vi "Plus minus conditional.vi"(8 "Percent Floor":dbl=2.0, 9 "Actual Number":dbl, 10 "Target":dbl, 11 "Percent ceiling":dbl=2.0) -> (0 "Below":bool, 2 "Either":bool, 3 "Above":bool)   [LabVIEW 2012]
doc: "This VI check to see if a number is above or below a certain percent."
panel:
  out "min":dbl
  out "max":dbl
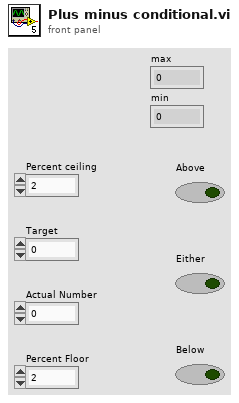
[diagram p1: front panel]
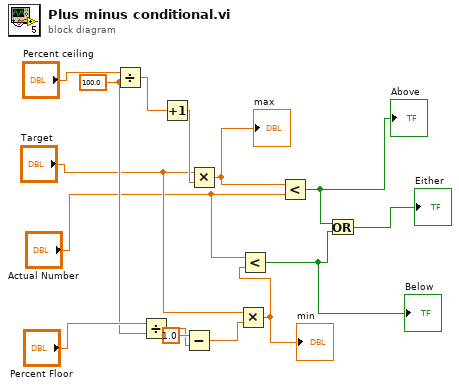
[diagram p0: block diagram]
diagram:
  w13 = 100.0 ("y")
  n1 = Divide(x="Percent ceiling", y=w13) -> (x/y=w12:dbl)
  n2 = Divide(x="Percent Floor", y=w13) -> (x/y=w2:dbl)
  n3 = Increment(x=w12) -> (x+1=w11:dbl)
  n4 = Subtract(x=1.0, y=w2) -> (x-y=w1:dbl)
  n5 = Multiply(x="Target", y=w11) -> (x*y=w10:dbl)
  "max" <- w10
  n6 = Multiply(x="Target", y=w1) -> (x*y=w5:dbl)
  "min" <- w5
  n7 = Less?(x="Actual Number", y=w5) -> (x < y?=w4:bool)
  "Below" <- w4
  n8 = Less?(x=w10, y="Actual Number") -> (x < y?=w9:bool)
  "Above" <- w9
  n9 = Or(x=w9, y=w4) -> (x .or. y?=→"Either":bool)
